vi "Timing-Elapsed Time.vi"(4 "Start time (ms)":u32, 5 "error in (no error)":errorcluster) -> (1 "Elapsed time (ms)":u32)   [LabVIEW 2020]
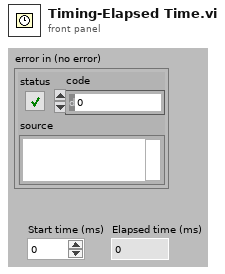
[diagram p1: front panel]
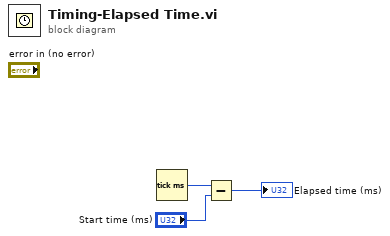
[diagram p0: block diagram]
diagram:
  n1 = Tick Count (ms)() -> (millisecond timer value=w3:u32)
  n2 = Subtract(x=w3, y="Start time (ms)") -> (x-y=→"Elapsed time (ms)":u32)
